vi "CANFD Init.vi"(8 "error in (no error)":errorcluster, 9 "pCanConfig":T1, 10 "CANIndex":u8, 11 "DevHandle":i32) -> (0 "error out":errorcluster, 1 "pCanConfig out":T1, 3 "function return":i32)   [LabVIEW 2010, in "usb2canfd.lvlib"]
doc: "int WINAPI CANFD_Init(int DevHandle, unsigned char CANIndex, CANFD_INIT_CONFIG *pCanConfig);"
uses:
  usb2canfd.lvlib
  examples/Labview/PublicFiles/USB2XXX.dll
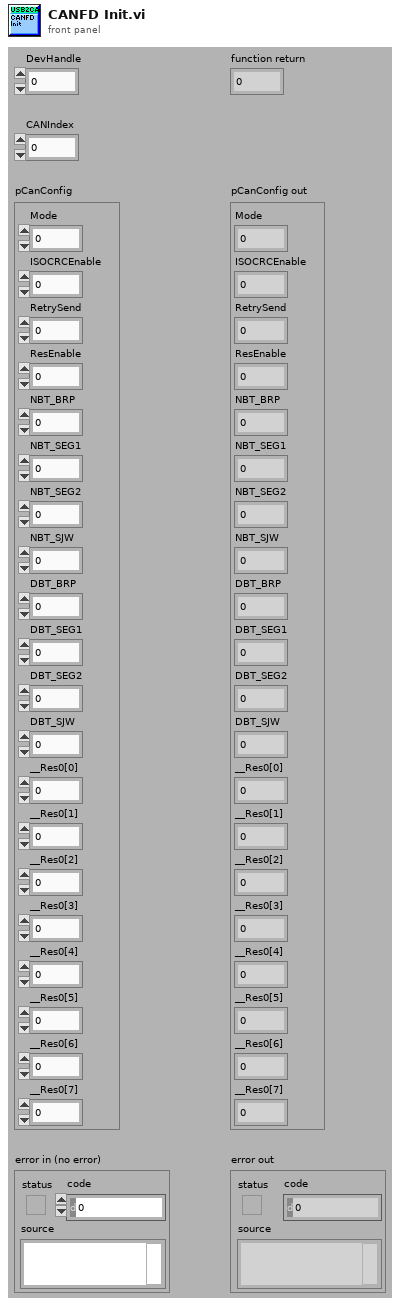
[diagram p1: front panel]
types:
  T1 = cluster{"Mode":u8, "ISOCRCEnable":u8, "RetrySend":u8, "ResEnable":u8, "NBT_BRP":u8, "NBT_SEG1":u8, "NBT_SEG2":u8, "NBT_SJW":u8, "DBT_BRP":u8, "DBT_SEG1":u8, "DBT_SEG2":u8, "DBT_SJW":u8, "__Res0[0]":u8, "__Res0[1]":u8, "__Res0[2]":u8, "__Res0[3]":u8, "__Res0[4]":u8, "__Res0[5]":u8, "__Res0[6]":u8, "__Res0[7]":u8}
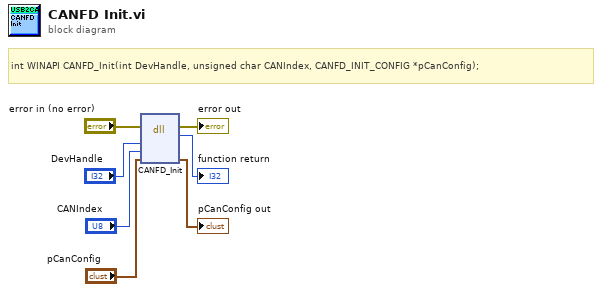
[diagram p0: block diagram]
diagram:
  # "int WINAPI CANFD_Init(int DevHandle, unsigned char CANIndex, CANFD_INIT_CONFIG *pCanConfig);"
  n1 = dll-call lib="E:/OtherWork/STM32/USB2XXX_Example/examples/Labview/PublicFiles/USB2XXX.*" fn="CANFD_Init"(error in="error in (no error)", "DevHandle"="DevHandle", "CANIndex"="CANIndex", "pCanConfig"="pCanConfig") -> (error out=→"error out":errorcluster, →"function return":i32, "pCanConfig"=→"pCanConfig out":T1)  [unwired: 4 in, 1 out]
